vi "Motor de Passo LabView Com Stepper.vi"() -> ()   [LabVIEW 2010]
uses:
  <vilib>/LabVIEW Interface for Arduino/LabVIEW Interface for Arduino.lvlib
panel:
  in  "Sentido":bool
  out "XY Graph":cluster{"Y":dbl[], "Y":dbl[]}[](graph)
  in  "Passos por Segundo":dbl
  in  "Número de Passos Para se Mover":i16
  in  "Parar":bool
  in  "Pinos do Motor de Passo":u8[](array[numeric])=[2, 3]
  # "Passo"
  # "Direção"
  # "48"
  # "1 = 390s pra 1 rot"
  # "Anti-Horário"
  # "Horário"
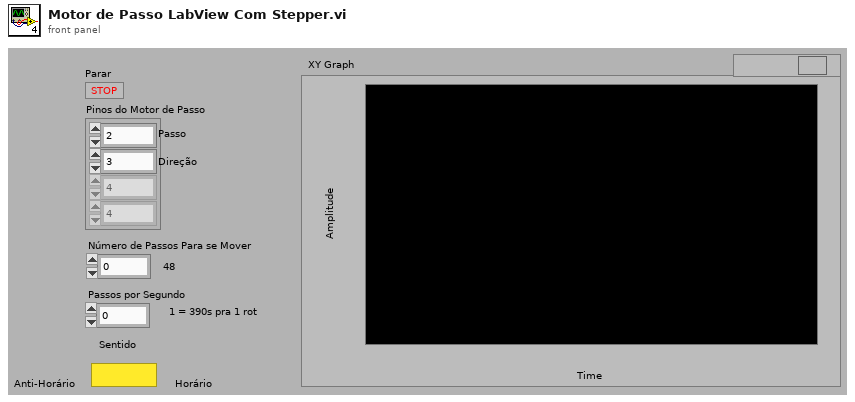
[diagram p1: front panel]
types:
  T1 = typedef "LabVIEW Interface for Arduino.lvlib/Arduino Resource.ctl" = cluster{"VISA resource":refnum<visa-resource-name>, "Board Type":T2, "Connection Type":enum8{"USB / Serial"}, "Bytes Per Packet (15)":u8}
  T2 = typedef "LabVIEW Interface for Arduino.lvlib/Board Type.ctl" = enum16{"Uno", "Dimuelanove w/Atmega 328", "Mega 2560"}
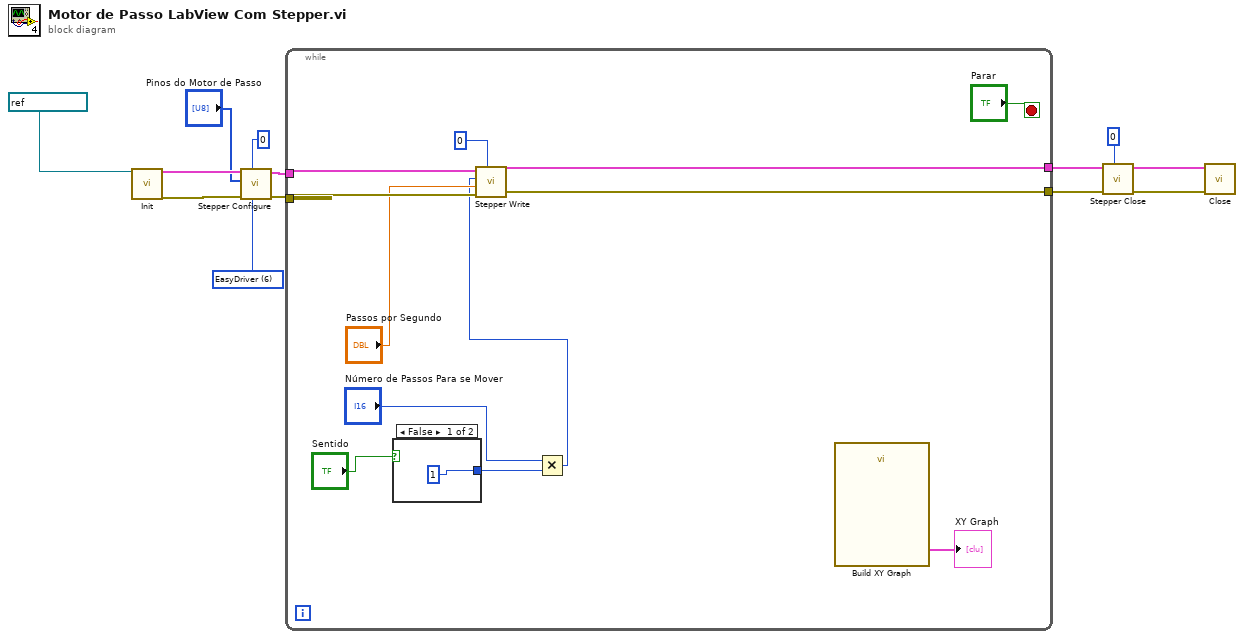
[diagram p0: block diagram]
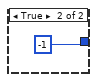
[diagram p2: hidden frame]
diagram:
  w11 = u8 6 items=["2 Wire (Pulse & Direction)"=1, "2 Wire"=2, "4 Wire"=4, "EasyDriver"=6, "AF Motor Shield (Stepper 1 & 2 Only)"=5] ("Control Method")
  n1 = call <vilib>:"Init.vi"("VISA resource"=refnum<visa-resource-name> "COM4") -> ("Arduino Resource"=w12:T1, "error out"=w10:errorcluster)  [unwired: 17 in]
  n2 = call <vilib>:"Stepper Configure.vi"("Control Method"=w11, "Stepper #"=u8 0, "error in"=w10, "Stepper Pins"="Pinos do Motor de Passo", "Arduino Resource"=w12) -> ("error out"=w7:errorcluster, "Arduino Resource Out"=w8:T1)  [unwired: 5 in]
  n3 = while {
    tunnel: w8 -> [w23]
    tunnel: w7 -> [w22]
    tunnel: [w21] -> w1
    tunnel: [w24] -> w5
    stop <- "Parar" stop-if-true
    n4 = case shown="False" "Sentido" {
      tunnel: [1 -1] -> w16
      frame False {
      }
      frame True {
      }
    }
    n5 = Multiply(x="Número de Passos Para se Mover", y=w16) -> (x*y=w14:i32)
    n6 = call <vilib>:"Stepper Write.vi"("Stepper #"=u8 0, "error in"=w22, "Set Speed (Steps per Second)"="Passos por Segundo", "# of Steps to Move"=w14, "Arduino Resource"=w23) -> ("error out"=w24:errorcluster, "Arduino Resource Out"=w21:T1)  [unwired: 5 in]
    n7 = call "Build XY Graph"() -> ("XY Graph"=→"XY Graph":cluster{"Y":dbl[], "Y":dbl[]}[])  [unwired: 5 in, 6 out]
  }
  n8 = call <vilib>:"Stepper Close.vi"("Stepper #"=u8 0, "error in"=w5, "Arduino Resource"=w1) -> ("error out"=w3:errorcluster, "Arduino Resource Out"=w2:T1)  [unwired: 7 in]
  n9 = call <vilib>:"Close.vi"("Arduino Resource"=w2, "error in"=w3) -> ()  [unwired: 13 in, 1 out]
